vi "initialize imu dmp.vi"(0 "data":T1, 1 "accel_fsr":u32(ring) items=["A_FSR_2G", "A_FSR_4G", "A_FSR_8G", "A_FSR_16G"], 2 "gyro_fsr":u32(ring) items=["G_FSR_250DPS", "G_FSR_500DPS", "G_FSR_1000DPS", "G_FSR_2000DPS"], 3 "gyro_dlpf":u32(ring) items=["GYRO_DLPF_OFF", "GYRO_DLPF_184", "GYRO_DLPF_92", "GYRO_DLPF_41", "GYRO_DLPF_20", "GYRO_DLPF_10", "GYRO_DLPF_5"], 4 "accel_dlpf":u32(ring) items=["ACCEL_DLPF_OFF", "ACCEL_DLPF_184", "ACCEL_DLPF_92", "ACCEL_DLPF_41", "ACCEL_DLPF_20", "ACCEL_DLPF_10", "ACCEL_DLPF_5"], 5 "enable_magnetometer":i32, 6 "dmp_sample_rate":i32, 7 "error in (no error)":errorcluster, 8 "orientation":u32(ring)=136 items=["ORIENTATION_Z_UP"=136, "ORIENTATION_Z_DOWN"=396, "ORIENTATION_X_UP"=14, "ORIENTATION_X_DOWN"=266, "ORIENTATION_Y_UP"=112, "ORIENTATION_Y_DOWN"=336], 9 "compass_mix_factor":i32, 10 "dmp_interrupt_priority":i32, 11 "show_warnings":i32) -> (20 "data out":T1, 21 "function return":i32, 27 "error out":errorcluster)   [LabVIEW 2014, in "test_IMU.lvlib"]
doc: "int initialize_imu_dmp(imu_data_t *data, imu_config_t conf);"
uses:
  <userlib>/test_IMU/test_IMU.lvlib
  Users/ktalke/Documents/Updated Header File/6.18.16/Compiled SO -schroot/robotics_cape.so
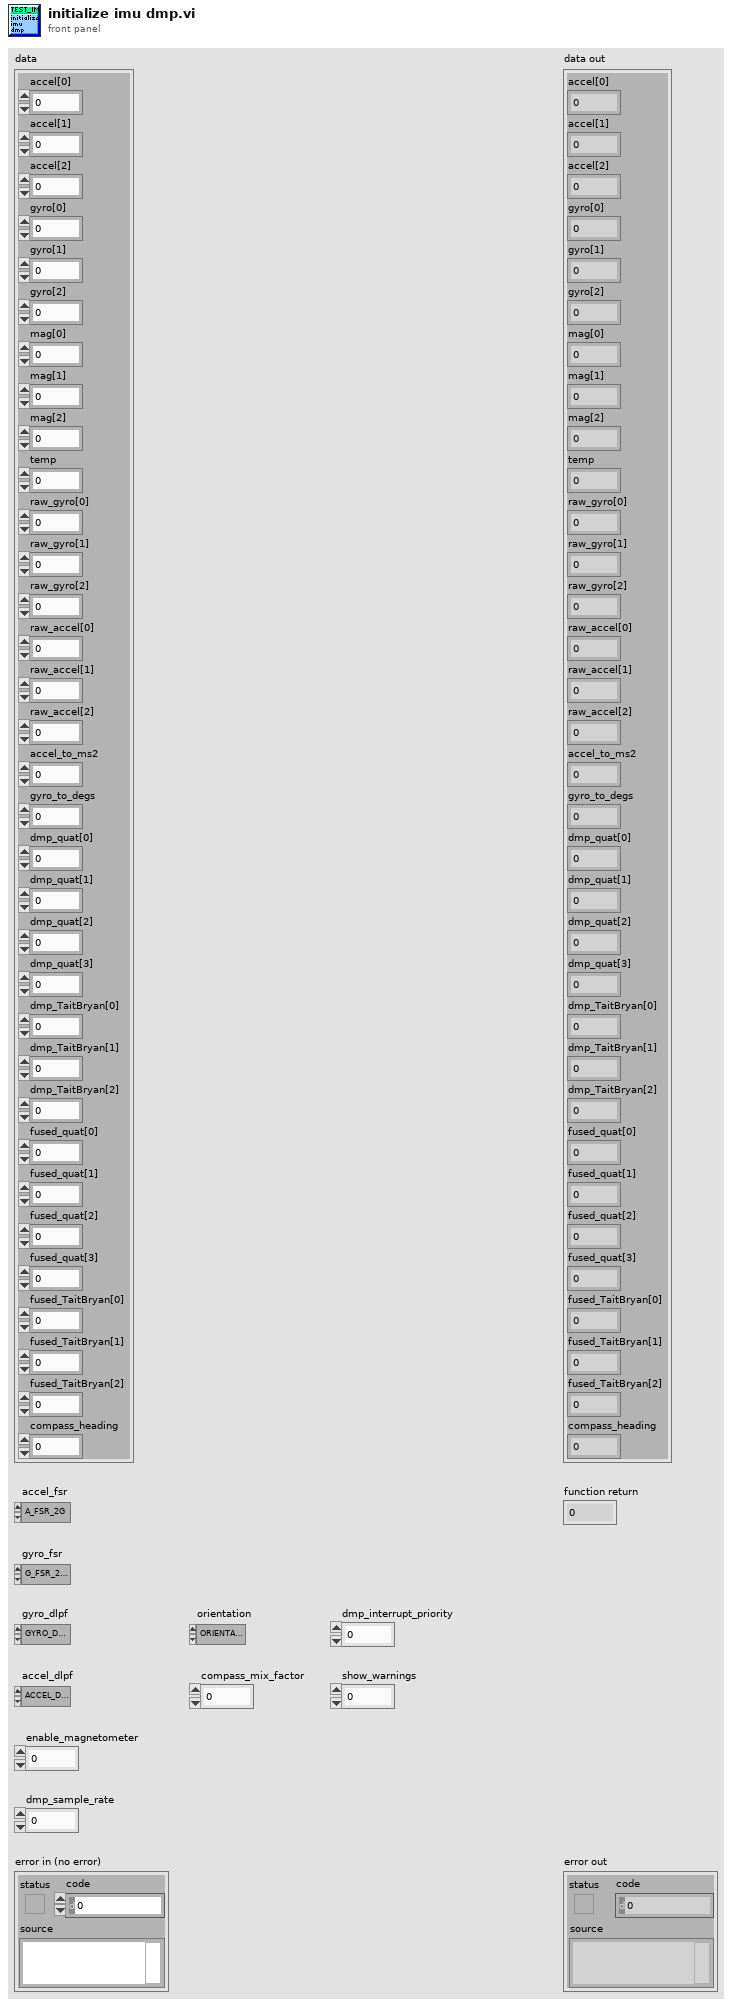
[diagram p1: front panel]
types:
  T1 = cluster{"accel[0]":sgl, "accel[1]":sgl, "accel[2]":sgl, "gyro[0]":sgl, "gyro[1]":sgl, "gyro[2]":sgl, "mag[0]":sgl, "mag[1]":sgl, "mag[2]":sgl, "temp":sgl, "raw_gyro[0]":i16, "raw_gyro[1]":i16, "raw_gyro[2]":i16, "raw_accel[0]":i16, "raw_accel[1]":i16, "raw_accel[2]":i16, "accel_to_ms2":sgl, "gyro_to_degs":sgl, "dmp_quat[0]":sgl, "dmp_quat[1]":sgl, "dmp_quat[2]":sgl, "dmp_quat[3]":sgl, "dmp_TaitBryan[0]":sgl, "dmp_TaitBryan[1]":sgl, "dmp_TaitBryan[2]":sgl, "fused_quat[0]":sgl, "fused_quat[1]":sgl, "fused_quat[2]":sgl, "fused_quat[3]":sgl, "fused_TaitBryan[0]":sgl, "fused_TaitBryan[1]":sgl, "fused_TaitBryan[2]":sgl, "compass_heading":sgl}
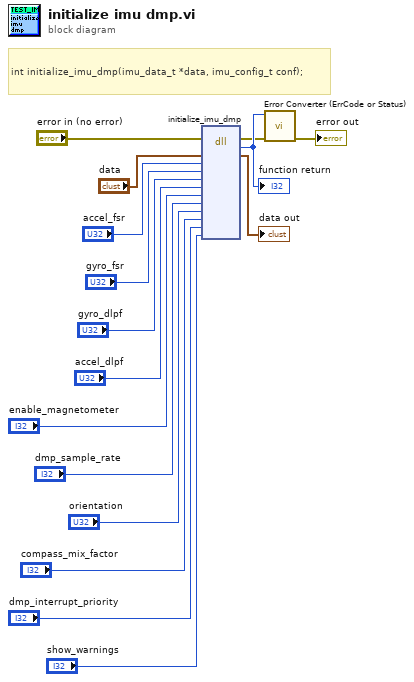
[diagram p0: block diagram]
diagram:
  # "int initialize_imu_dmp(imu_data_t *data, imu_config_t conf);"
  n1 = dll-call lib="C:/Users/ktalke/Documents/Updated Header File/6.18.16/Compiled SO -schroot/robotics_cape.so" fn="initialize_imu_dmp"(error in="error in (no error)", "data"="data", "accel_fsr"="accel_fsr", "gyro_fsr"="gyro_fsr", "gyro_dlpf"="gyro_dlpf", "accel_dlpf"="accel_dlpf", "enable_magnetometer"="enable_magnetometer", "dmp_sample_rate"="dmp_sample_rate", "orientation"="orientation", "compass_mix_factor"="compass_mix_factor", "dmp_interrupt_priority"="dmp_interrupt_priority", "show_warnings"="show_warnings") -> (error out=w2:errorcluster, w16:i32, "data"=→"data out":T1)  [unwired: 12 in, 1 out]
  "function return" <- w16
  n2 = call <userlib>:"Error Converter (ErrCode or Status).vi"("error in (no error)"=w2, "error code"=w16) -> ("error out"=→"error out":errorcluster)  [unwired: 9 in]
